vi "test Compile RaF Communication.vi"(8 "error in (no error)":errorcluster, 11 "TestCase in":refnum<class "Routing and Faulting Compile Unit Tests.lvclass">) -> (0 "error out":errorcluster, 3 "TestCase out":refnum<class "Routing and Faulting Compile Unit Tests.lvclass">)   [LabVIEW 2020, in "Routing and Faulting Compile Unit Tests.lvclass"]
uses:
  Routing and Faulting Compile Unit Tests.lvclass
  Shared/Communication Configuration.ctl
  Routing and Faulting Compile Unit Tests.lvclass/Routing and Faulting Compile Unit Tests.ctl
  Scripting/Routing and Faulting Scripting.lvlib
  System Explorer/Routing and Faulting System Explorer.lvlib
  Shared/Routing and Faulting Shared.lvlib
panel:
  out "Communication Configuration":T1
  in  "Save?":bool
  out "Output Filename":string
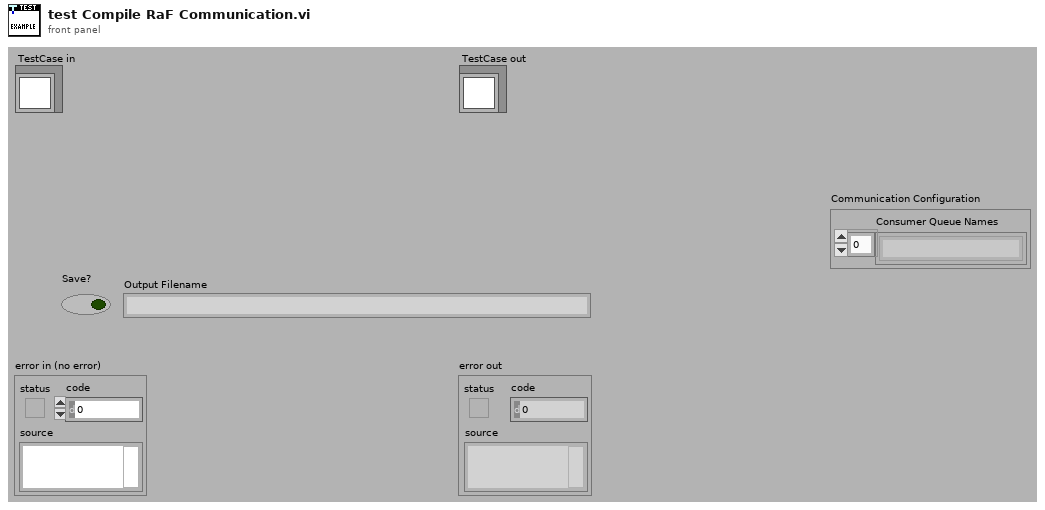
[diagram p1: front panel]
types:
  T1 = typedef "Routing and Faulting Shared.lvlib/Communication Configuration.ctl" = cluster{"Consumer Queue Names":string[]}
  T2 = typedef "Custom Device API.lvlib/Custom Device Item Ref.ctl" = u64
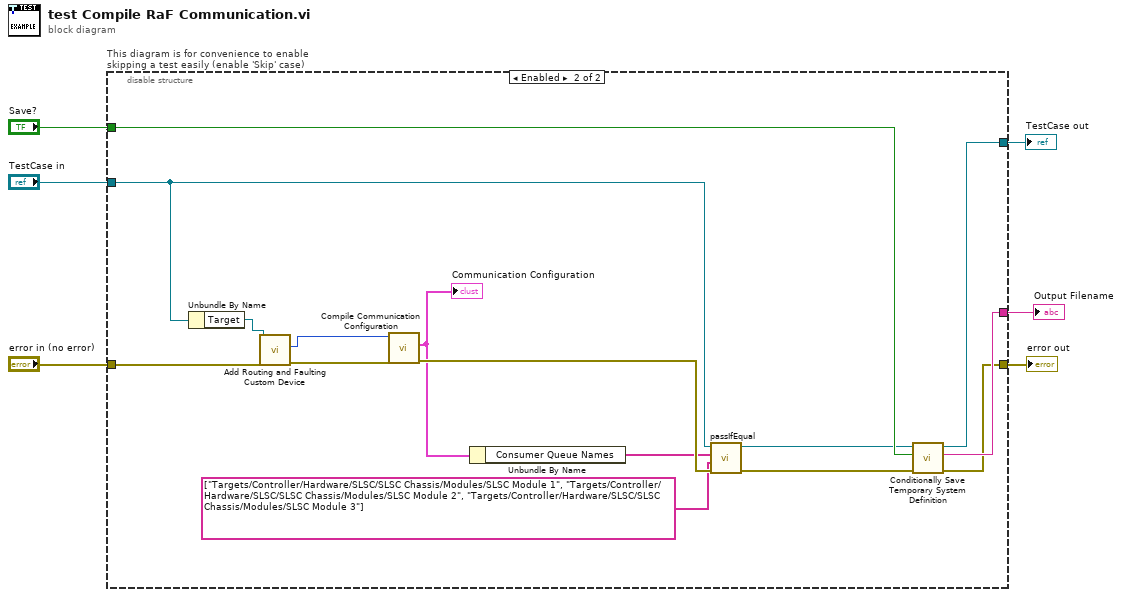
[diagram p0: block diagram]
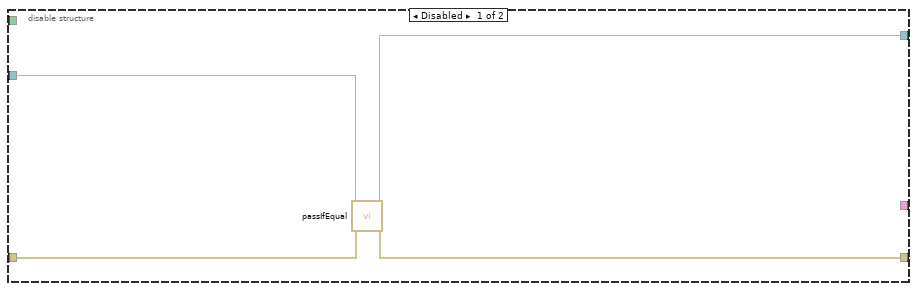
[diagram p2: hidden frame]
diagram:
  n1 = disable-structure "This diagram is for convenience to enable skipping a test easily (enable 'Skip' case)" shown="Enabled" {
    disable-tunnel: "TestCase in" -> [w10 w20]
    disable-tunnel: [w9 w22] -> w3
    disable-tunnel: [w8 w18] -> w5
    disable-tunnel: "error in (no error)" -> [w7 w24]
    disable-tunnel: "Save?" -> [_ w23]
    disable-tunnel: [_ w21] -> w1
    frame Disabled {
      n2 = call-dynamic "passIfEqual.vi"("error in (no error)"=w7, "TestCase in"=w10) -> ("error out"=w8:errorcluster, "TestCase out"=w9:refnum<class "Routing and Faulting Compile Unit Tests.lvclass">)  [unwired: 8 in]
    }
    frame Enabled {
      n3 = Unbundle By Name(w20) -> ("Target"=w25:refnum<k24>)
      n4 = call "Add Routing and Faulting Custom Device.vi"("error in"=w24, "target in"=w25) -> ("error out"=w16:errorcluster, "routing and faulting custom device"=w15:T2)  [unwired: 7 in, 1 out]
      n5 = call "Compile Communication Configuration.vi"("error in (no error)"=w16, "Device Ref in"=w15) -> ("error out"=w14:errorcluster, "Communication Configuration"=w11:T1)  [unwired: 7 in, 1 out]
      "Communication Configuration" <- w11
      n6 = Unbundle By Name(w11) -> ("Consumer Queue Names"=w13:string[])
      n7 = call-dynamic "passIfEqual.vi"("error in (no error)"=w14, "y"=string[] ["Targets/Controller/Hardware/SLSC/SLSC Chassis/Modules/SLSC Module 1", "Targets/Controller/Hardware/SLSC/SLSC Chassis/Modules/SLSC Module 2", "Targets/Controller/Hardware/SLSC/SLSC Chassis/Modules/SLSC Module 3"] ("Consumer Queue Names"), "x"=w13, "TestCase in"=w20) -> ("error out"=w17:errorcluster, "TestCase out"=w19:refnum<class "Routing and Faulting Compile Unit Tests.lvclass">)  [unwired: 6 in]
      n8 = call "Conditionally Save Temporary System Definition.vi"("error in (no error)"=w17, "Save?"=w23, "TestCase in"=w19) -> ("error out"=w18:errorcluster, "filename"=w21:string, "TestCase out"=w22:refnum<class "Routing and Faulting Compile Unit Tests.lvclass">)  [unwired: 6 in]
    }
  }
  "error out" <- w5
  "TestCase out" <- w3
  "Output Filename" <- w1
